vi "Get Bundler Items Displayed.vi"(11 "Affected Items":T2) -> (3 "Displayed Items":T1[](array[typedef]))   [LabVIEW 2023]
doc: "Get input or outpur terminals displayed from a named bundler or unbundler. This is used for the dialog to remove and rearrange those items."
uses:
  top/BundleMagic.ctl
  Cluster Element Description.ctl
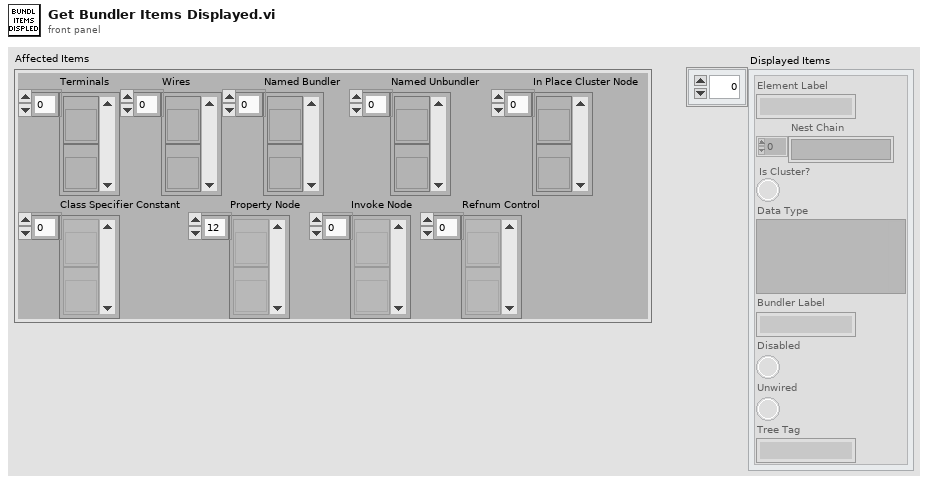
[diagram p1: front panel]
types:
  T1 = typedef "Cluster Element Description.ctl" = cluster{"Element Label":string, "Nest Chain":string[], "Is Cluster?":bool, "Data Type":variant, "Bundler Label":string, "Disabled":bool, "Unwired":bool, "Tree Tag":string}
  T2 = typedef "BundleMagic.ctl" = cluster{"Terminals":refnum<vi>[], "Wires":refnum<vi>[], "Named Bundler":refnum<vi>[], "Named Unbundler":refnum<vi>[], "In Place Cluster Node":refnum<vi>[], "Class Specifier Constant":refnum<vi>[], "Property Node":refnum<vi>[], "Invoke Node":refnum<vi>[], "Refnum Control":refnum<vi>[]}
  T3 = enum16{"Named Bundler", "Named Unbundler", "In Place", "None"}
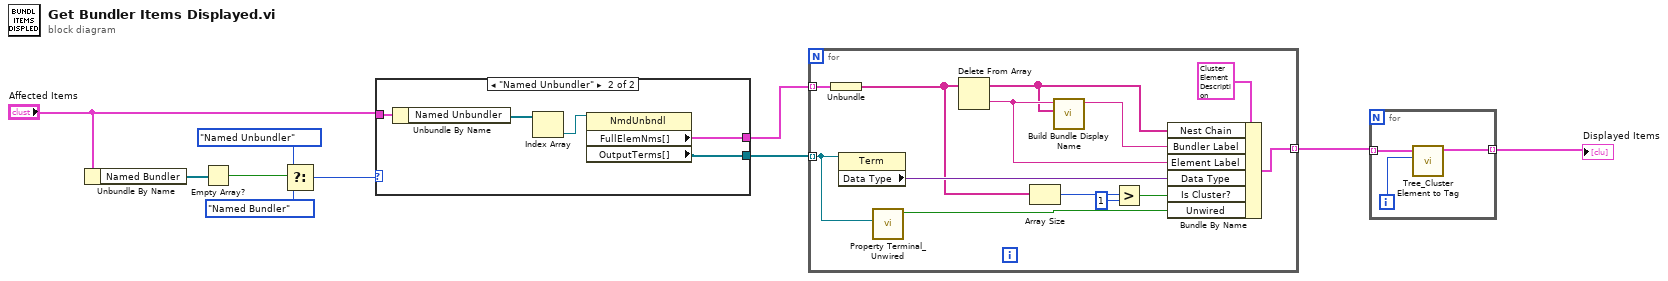
[diagram p0: block diagram]
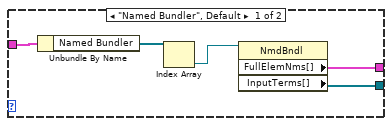
[diagram p2: hidden frame]
diagram:
  n1 = Unbundle By Name("Affected Items") -> ("Named Bundler"=w6:refnum<vi>[])
  n2 = Empty Array?(array=w6) -> (empty?=w5:bool)
  n3 = Select(t=T3."Named Unbundler" ("Bundler Type"), s=w5, f=T3."Named Bundler" ("Bundler Type")) -> (s? t:f=w4:T3)
  n4 = case shown="\"Named Unbundler\"" w4 {
    tunnel: [w15 w16] -> w9
    tunnel: [w14 w20] -> w10
    tunnel: "Affected Items" -> [w13 w19]
    frame "Named Bundler", Default {
      n5 = Unbundle By Name(w13) -> ("Named Bundler"=w12:refnum<vi>[])
      n6 = Index Array(array=w12) -> (element=w11:refnum<vi>)  [unwired: 1 in]
      n7 = property class="NmdBndl"(reference=w11) -> ("FullElemNms[]"=w15:cluster{string[]}[], "InputTerms[]"=w14:refnum<vi>[])  [unwired: 1 in, 2 out]
    }
    frame "Named Unbundler" {
      n8 = Unbundle By Name(w19) -> ("Named Unbundler"=w18:refnum<vi>[])
      n9 = Index Array(array=w18) -> (element=w17:refnum<vi>)  [unwired: 1 in]
      n10 = property class="NmdUnbndl"(reference=w17) -> ("FullElemNms[]"=w16:cluster{string[]}[], "OutputTerms[]"=w20:refnum<vi>[])  [unwired: 1 in, 2 out]
    }
  }
  n11 = for {
    tunnel: w10 -> [w22] mode=indexing
    tunnel: w9 -> [w30] mode=indexing
    tunnel: [w31] -> w2 mode=indexing
    n12 = Unbundle(w30) -> (w23:string[])
    n13 = property class="Term"(reference=w22) -> ("Data Type"=w32:variant)  [unwired: 1 in, 2 out]
    n14 = call "Property Terminal_Unwired.vi"("Term Refnum"=w22) -> ("Unwired"=w21:bool)  [unwired: 8 in, 2 out]
    n15 = Delete From Array(array=w23) -> (deleted portion=w29:string, array with subset deleted=w25:string[])  [unwired: 2 in]
    n16 = Array Size(array=w23) -> (size(s)=w28:i32)
    n17 = call "Build Bundle Display Name.vi"("Nest Chain"=w25, "Element Label"=w29) -> ("Bundle display name"=w24:string)  [unwired: 9 in]
    n18 = Greater?(x=w28, y=1) -> (0:w26:bool)
    n19 = Bundle By Name(cluster=T1 {"Element Label"="", "Nest Chain"=[], "Is Cluster?"=FALSE, "Data Type"=variant, "Bundler Label"="", "Disabled"=FALSE, "Unwired"=FALSE, "Tree Tag"=""} ("Cluster"), "Nest Chain"=w25, "Bundler Label"=w24, "Element Label"=w29, "Data Type"=w32, "Is Cluster?"=w26, "Unwired"=w21) -> (w31:T1)
  }
  n20 = for {
    tunnel: w2 -> [w36] mode=indexing
    tunnel: [w34] -> w1 mode=indexing
    i -> [w35]
    n21 = call "Tree_Cluster Element to Tag.vi"("Index"=w35, "Cluster Element Data"=w36) -> ("Cluster Element Data Out"=w34:T1)  [unwired: 8 in, 1 out]
  }
  "Displayed Items" <- w1
